vi "Corridor Switch Turn.vi"() -> ()   [LabVIEW 2017]
uses:
  Support Code/Starting Position.ctl
  <vilib>/Rock Robotics/WPI/Framework/Command Status Info.ctl
  <vilib>/Rock Robotics/WPI/Framework/Completion Status.ctl
  <vilib>/Rock Robotics/WPI/Framework/Completion Notifier.ctl
panel:
  out "Command Info Out":T1
  in  "Command Info In":T1
  in  "Starting Position":T4
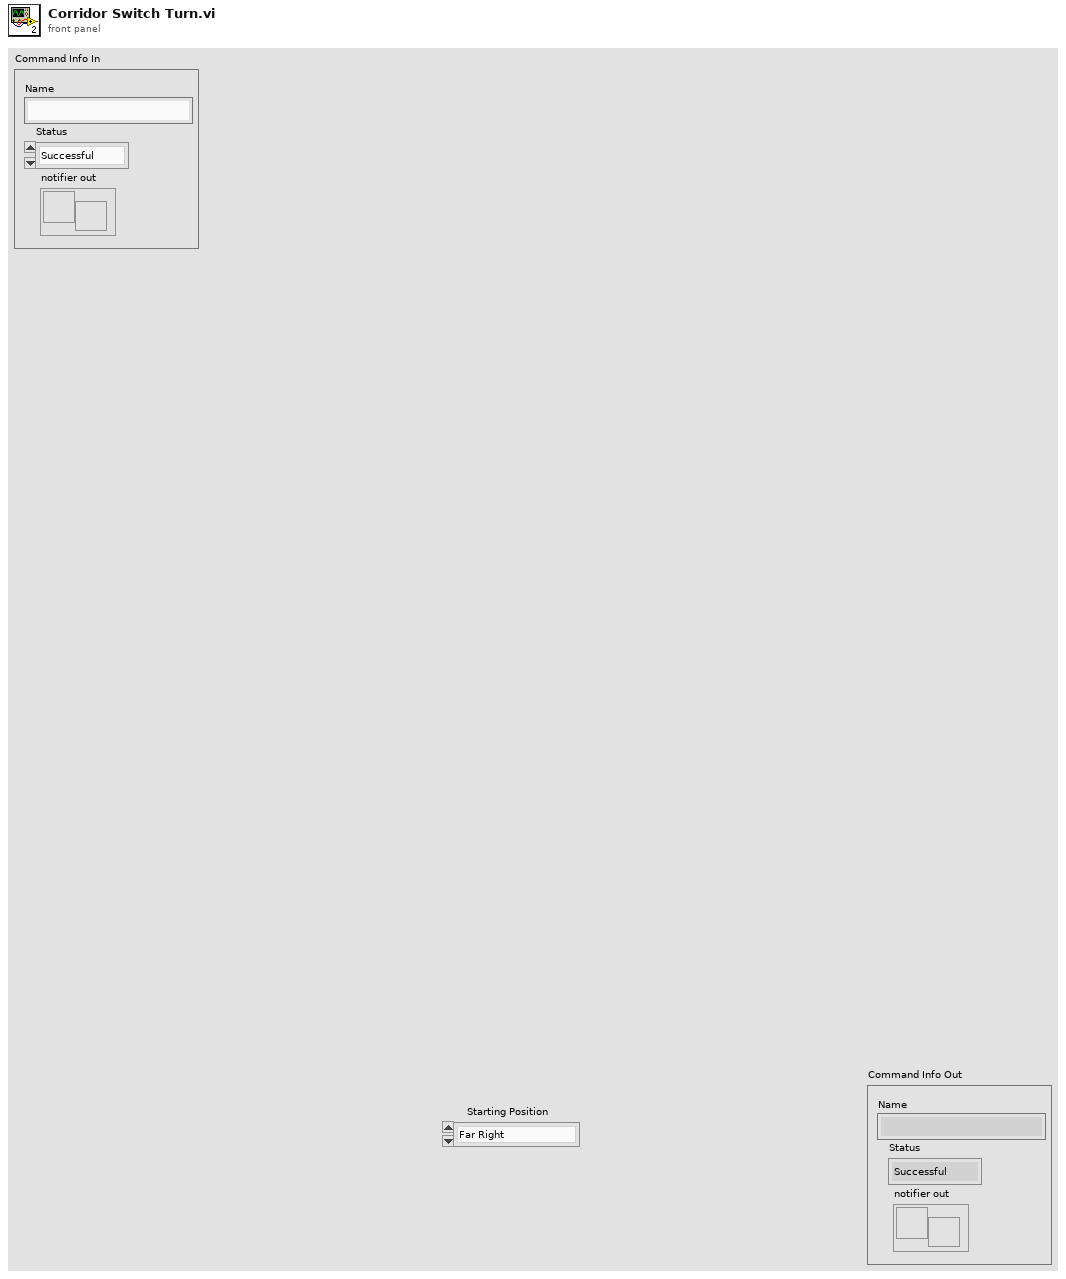
[diagram p1: front panel]
types:
  T1 = typedef "Command Status Info.ctl" = cluster{"Name":string, "Status":T2, "notifier out":T3}
  T2 = typedef "Completion Status.ctl" = enum16{"Successful", "Aborted", "Incomplete"}
  T3 = typedef "Completion Notifier.ctl" = refnum<notifier>
  T4 = typedef "Starting Position.ctl" = enum16{"Far Right", "Far Left"}
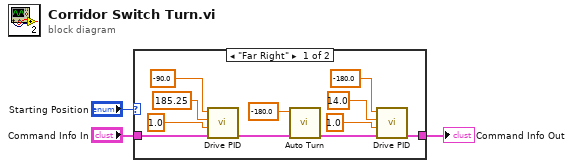
[diagram p0: block diagram]
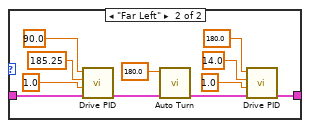
[diagram p2: hidden frame]
diagram:
  n1 = case shown="\"Far Right\"" "Starting Position" {
    tunnel: "Command Info In" -> [w13 w23]
    tunnel: [w4 w15] -> w1
    frame "Far Right" {
      n2 = call "Drive PID.vi"("Command Info In"=w13, "Speed"=1.0, "Distance"=185.25, "Target Angle"=-90.0) -> ("Command Info Out"=w9:T1)  [unwired: 7 in]
      n3 = call "Auto Turn.vi"("Command Info In"=w9, "Target Angle"=-180.0) -> ("Command Info Out"=w5:T1)  [unwired: 9 in]
      n4 = call "Drive PID.vi"("Command Info In"=w5, "Speed"=1.0, "Distance"=14.0, "Target Angle"=-180.0) -> ("Command Info Out"=w4:T1)  [unwired: 7 in]
    }
    frame "Far Left" {
      n5 = call "Drive PID.vi"("Command Info In"=w23, "Speed"=1.0, "Distance"=185.25, "Target Angle"=90.0) -> ("Command Info Out"=w20:T1)  [unwired: 7 in]
      n6 = call "Auto Turn.vi"("Command Info In"=w20, "Target Angle"=180.0) -> ("Command Info Out"=w19:T1)  [unwired: 9 in]
      n7 = call "Drive PID.vi"("Command Info In"=w19, "Speed"=1.0, "Distance"=14.0, "Target Angle"=180.0) -> ("Command Info Out"=w15:T1)  [unwired: 7 in]
    }
  }
  "Command Info Out" <- w1
